vi "meetCriteria.vi"(8 "error in (no error)":errorcluster, 10 "Persons In":refnum<class "Person.lvclass">[](array[class]), 11 "OrCriteria in":refnum<class "OrCriteria.lvclass">) -> (0 "error out":errorcluster, 2 "Persons Out":refnum<class "Person.lvclass">[](array[class]), 3 "OrCriteria out":refnum<class "OrCriteria.lvclass">)   [LabVIEW 2018, in "OrCriteria.lvclass"]
uses:
  OrCriteria.lvclass
  Person Class/Person.lvclass
  OrCriteria.lvclass/OrCriteria.ctl
  Criteria Class/Criteria.lvclass
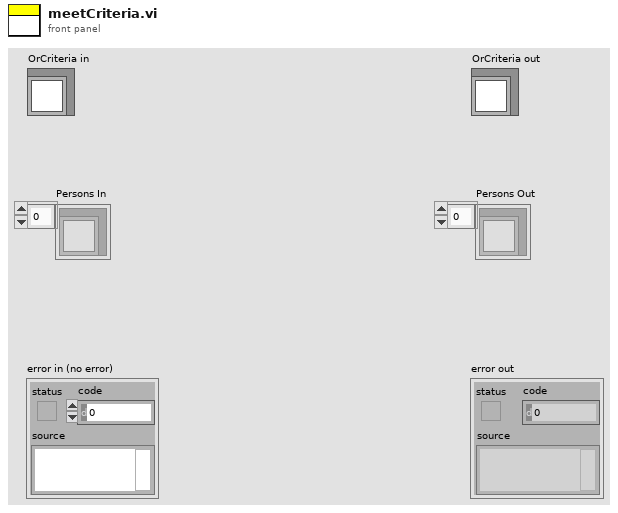
[diagram p1: front panel]
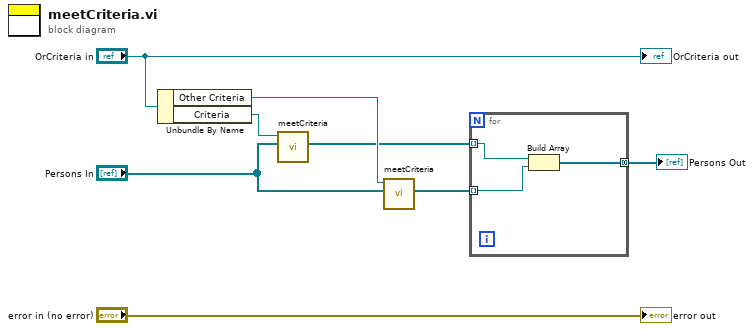
[diagram p0: block diagram]
diagram:
  n1 = Unbundle By Name("OrCriteria in") -> ("Other Criteria"=w5:refnum<class "Criteria.lvclass">, "Criteria"=w6:refnum<class "Criteria.lvclass">)
  n2 = call-dynamic "meetCriteria.vi"("Persons In"="Persons In", "Criteria in"=w6) -> ("Persons Out"=w2:refnum<class "Person.lvclass">[])  [unwired: 7 in, 2 out]
  n3 = call-dynamic "meetCriteria.vi"("Persons In"="Persons In", "Criteria in"=w5) -> ("Persons Out"=w3:refnum<class "Person.lvclass">[])  [unwired: 7 in, 2 out]
  n4 = for {
    tunnel: w3 -> [w10] mode=indexing
    tunnel: w2 -> [w11] mode=indexing
    tunnel: [w9] -> w1 mode=concatenating
    n5 = Build Array(w11, w10) -> (w9:refnum<class "Person.lvclass">[])
  }
  "Persons Out" <- w1
  "error out" <- "error in (no error)"
  "OrCriteria out" <- "OrCriteria in"
